vi "sub_main_cpu-memroy_usage.vi"(8 "error in":errorcluster) -> (0 "error out":errorcluster)   [LabVIEW 2019]
uses:
  Ctrl/cmd_common.ctl
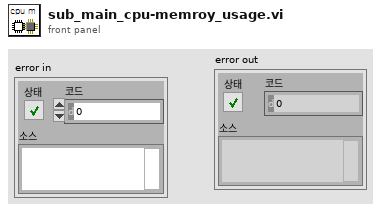
[diagram p1: front panel]
types:
  T1 = typedef "tools_system CPU Usage Ref.ctl" = cluster{"Query":u32, "Counter":u32}
  T2 = typedef "cmd_common.ctl" = enum16{"read", "write"}
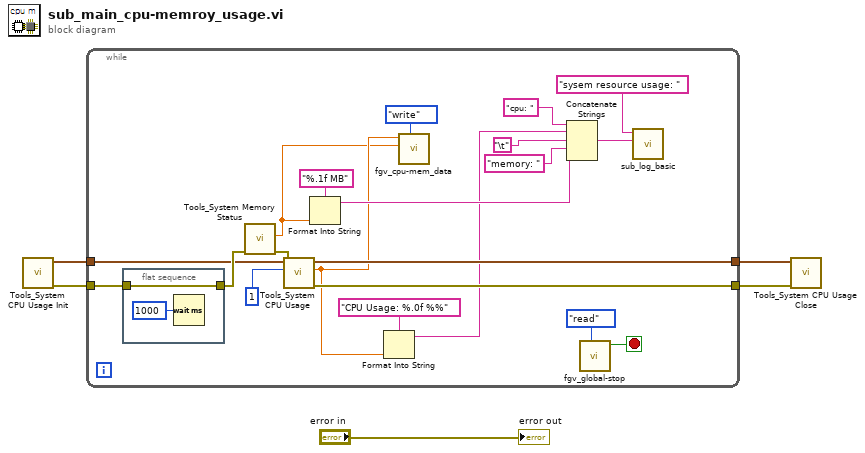
[diagram p0: block diagram]
diagram:
  n1 = call "Tools_System CPU Usage Init.vi"() -> ("error out"=w4:errorcluster, "CPU Usage Ref"=w3:T1)  [unwired: 10 in]
  n2 = while {
    tunnel: w4 -> [w17]
    tunnel: w3 -> [w16]
    tunnel: [w15] -> w2
    tunnel: [w14] -> w1
    stop <- w25 stop-if-true
    n3 = flat-sequence {
      tunnel: w17 -> [w27]
      tunnel: [w27] -> w18
      frame #0 {
        n4 = Wait (ms)(milliseconds to wait=u32 1000) -> ()  [unwired: 1 out]
      }
    }
    n5 = call "Tools_System Memory Status.vi"("error in (no error)"=w18) -> ("error out"=w19:errorcluster, "Free memory (MB)"=w7:dbl)  [unwired: 7 in, 2 out]
    n6 = call "Tools_System CPU Usage.vi"("error in"=w19, "index"=1, "CPU Usage Ref"=w16) -> ("error out"=w15:errorcluster, "CPU Usage (%)"=w8:dbl, "CPU Usage Ref"=w14:T1)  [unwired: 6 in]
    n7 = Format Into String(format string="%.1f MB", w7) -> (resulting string=w11:string)  [unwired: 2 in, 1 out]
    n8 = Format Into String(format string="CPU Usage: %.0f %%", w8) -> (resulting string=w10:string)  [unwired: 2 in, 1 out]
    n9 = call "fgv_cpu-mem_data.vi"("cmd"=cmd_common."write", "memory"=w7, "cpu"=w8) -> ()  [unwired: 7 in, 2 out]
    n10 = Concatenate Strings("cpu: " ("Title"), w10, "\t", "memory: " ("Title"), w11) -> (w24:string)
    n11 = call "fgv_global-stop.vi"("cmd"=enum16{"init", "stop", "read"}."read") -> ("val_out"=w25:bool)  [unwired: 10 in]
    n12 = call "sub_log_basic.vi"("desc"=w24, "Title"="sysem resource usage: ") -> ()  [unwired: 9 in, 1 out]
  }
  n13 = call "Tools_System CPU Usage Close.vi"("error in"=w2, "CPU Usage Ref"=w1) -> ()  [unwired: 9 in, 1 out]
  "error out" <- "error in"
